vi "Sensor information.vi"(8 "error in (no error)":errorcluster, 10 "Table":i32(listbox)) -> (0 "error in (no error) 2":errorcluster)   [LabVIEW 2015]
uses:
  Control Button/Exit.ctl
  Control Button/Save.ctl
  <vilib>/Utility/miscctls.llb/LVRowAndColumnTypeDef.ctl
  Control Button/Delete.ctl
panel:
  out "Row":i32
  out "subarray":string[](array[string])
  in  "Delete":T1
  in  "stop":T2
  in  "Save Button":T3
  out "Active Cell:Active Cell":T4
  # "Sensor Information"
  # "Sensor Name & Unit"
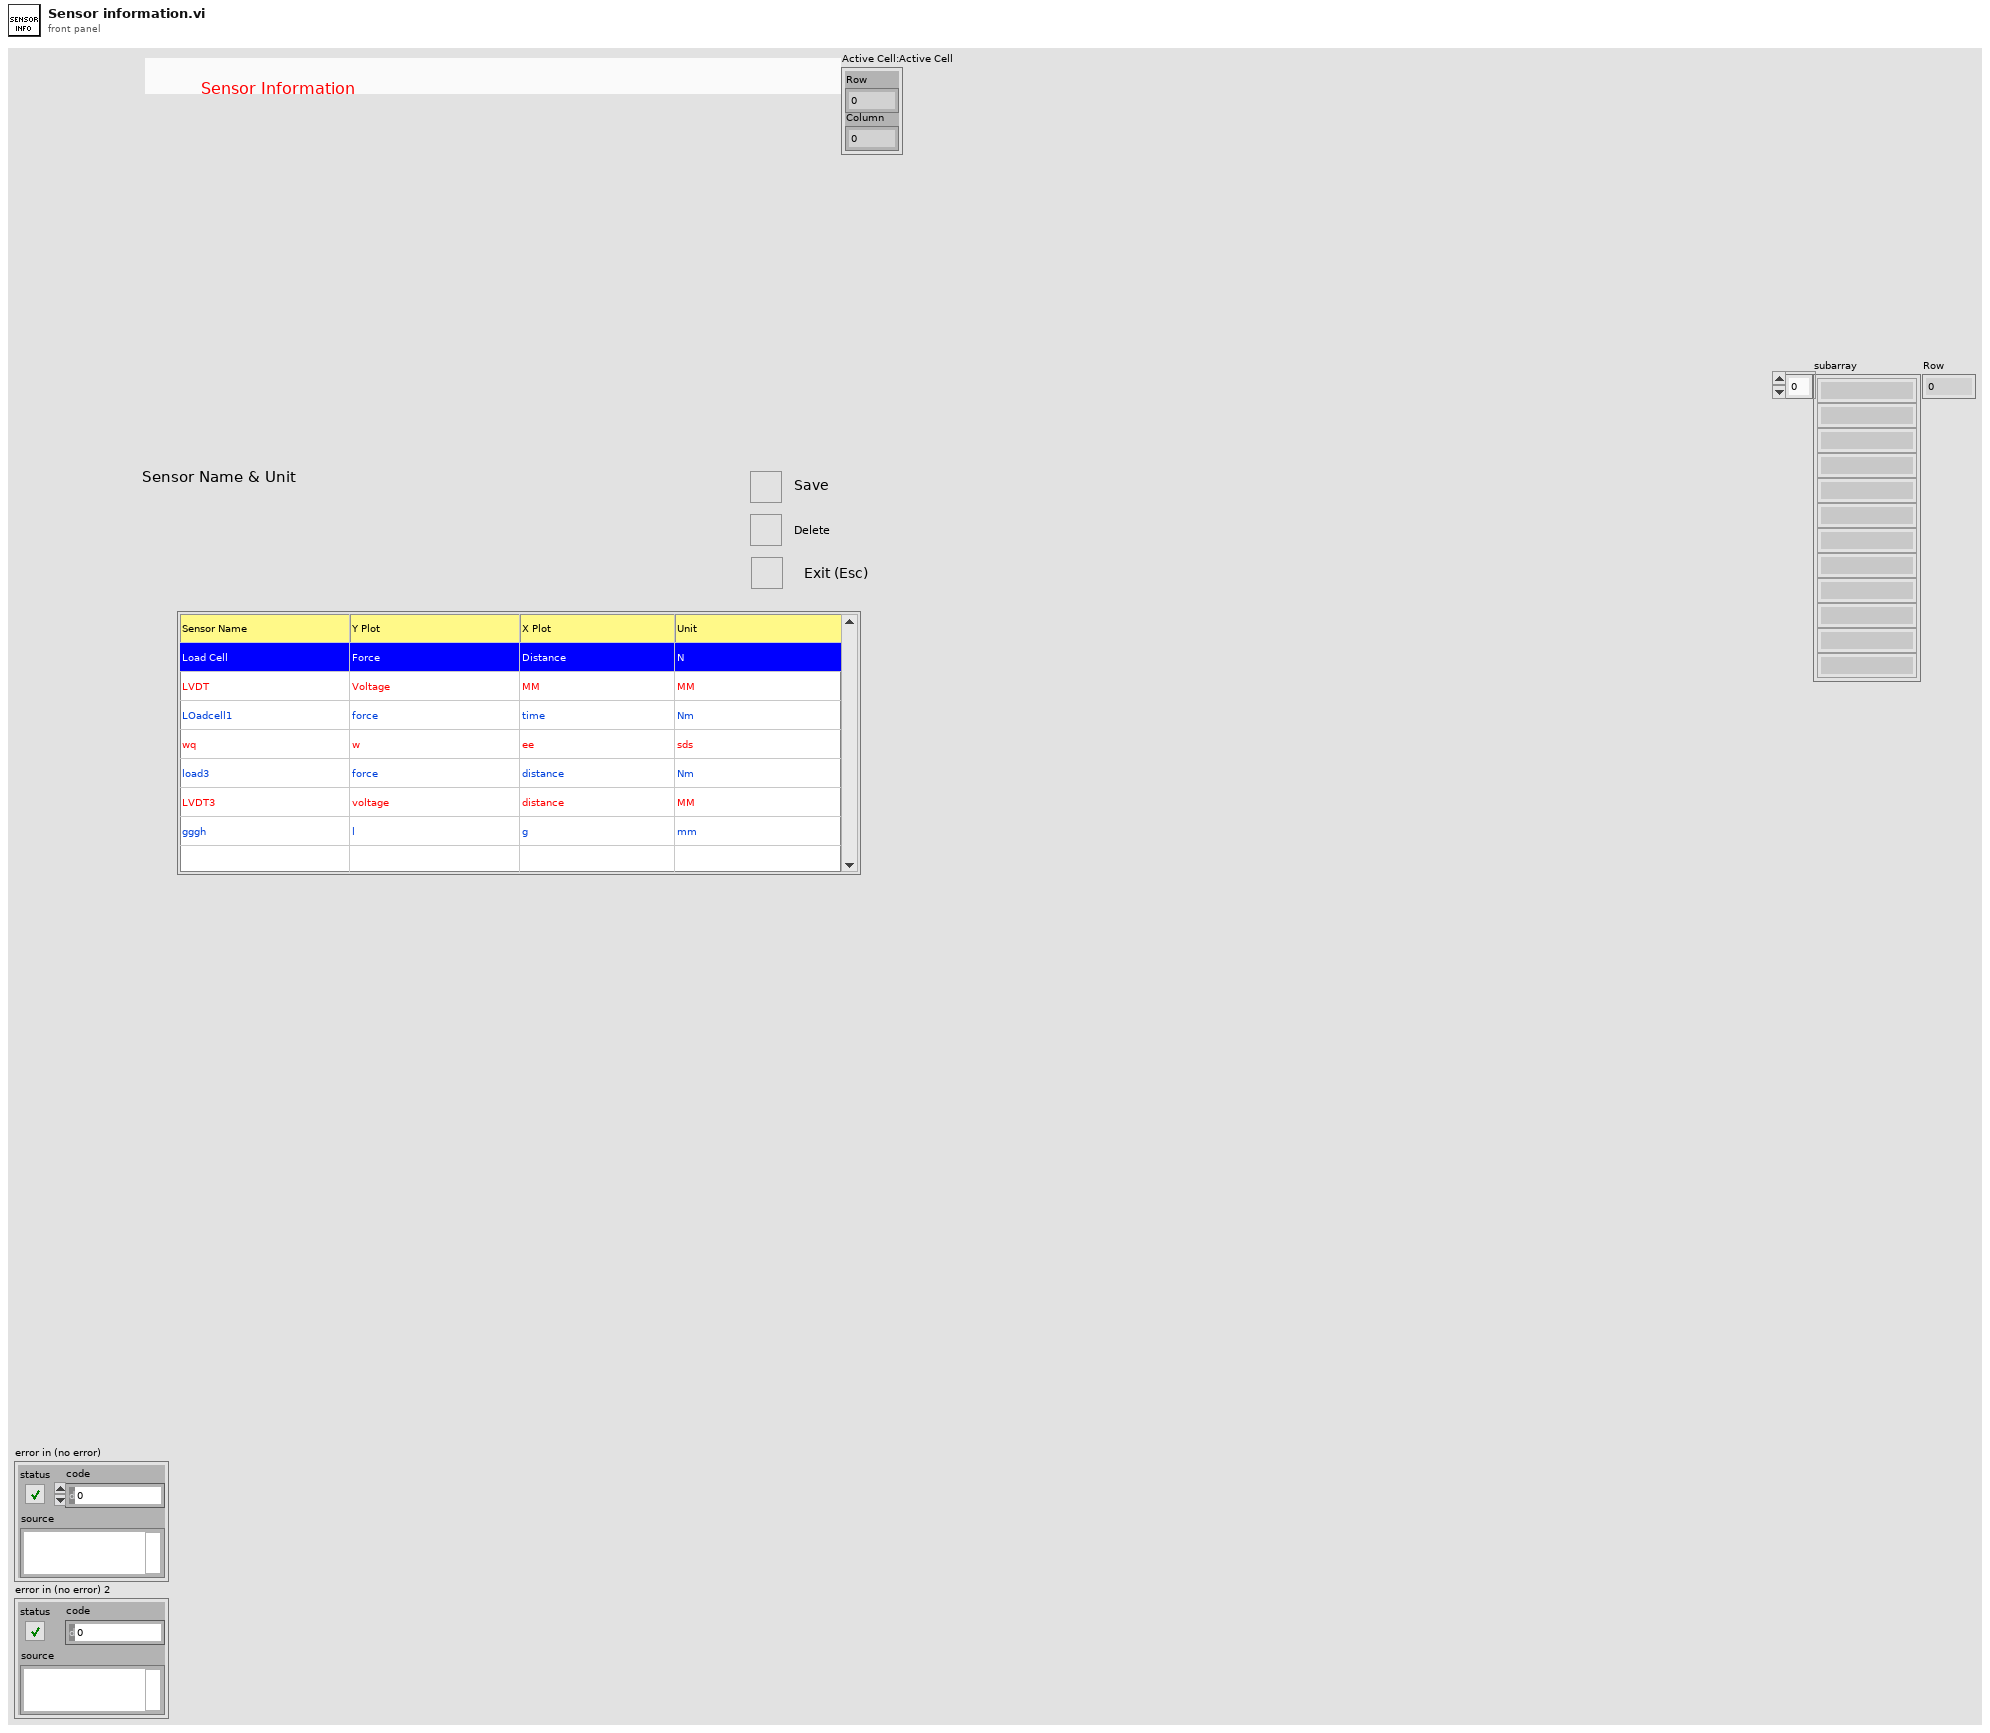
[diagram p1: front panel]
types:
  T1 = typedef "Delete.ctl" = bool
  T2 = typedef "Exit.ctl" = bool
  T3 = typedef "Save.ctl" = bool
  T4 = typedef "LVRowAndColumnTypeDef.ctl" = cluster{"Row":i32, "Column":i32}
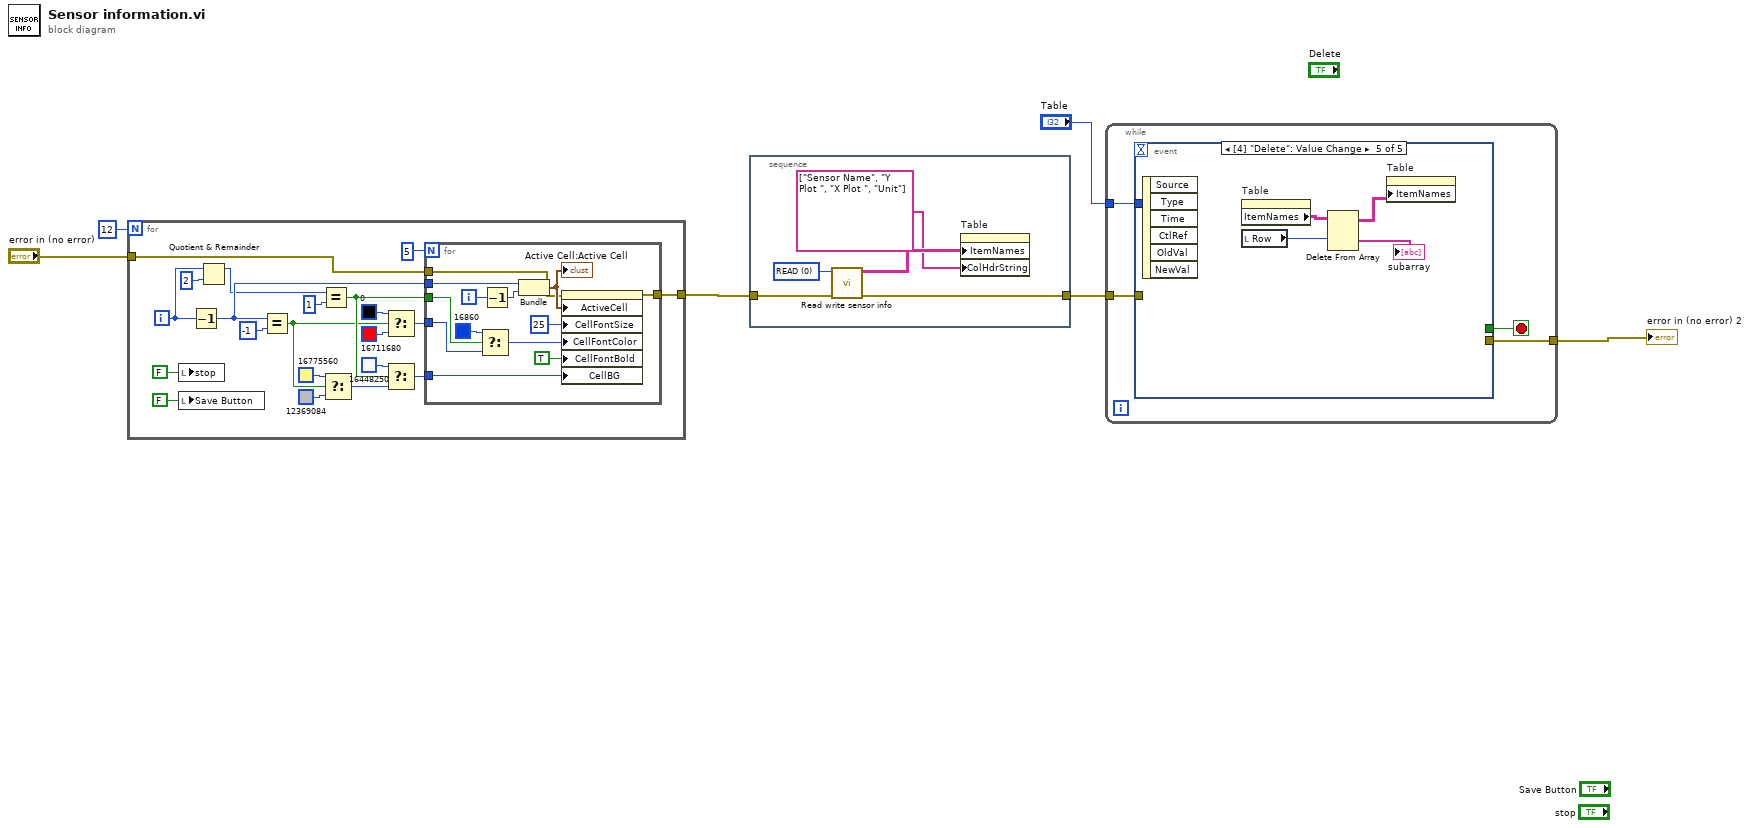
[diagram p0: block diagram]
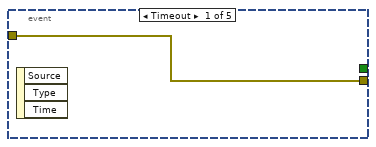
[diagram p2: hidden frame]
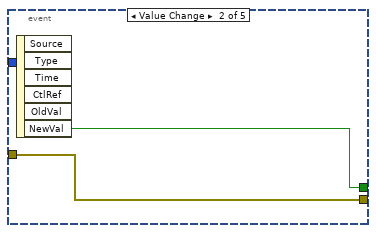
[diagram p3: hidden frame]
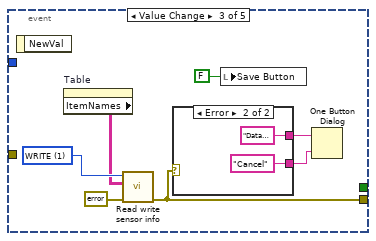
[diagram p4: hidden frame]
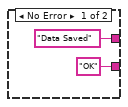
[diagram p5: hidden frame]
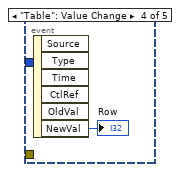
[diagram p6: hidden frame]
diagram:
  n1 = for {
    N: 12 -> [_]
    tunnel: [w10] -> w3
    tunnel: "error in (no error)" -> [w9]
    i -> [w22]
    n2 = local write "stop"(FALSE ("stop")) -> ()
    n3 = local write "Save Button"(FALSE ("Save Button")) -> ()
    n4 = Decrement(x=w22) -> (x-1=w20:i32)
    n5 = Quotient & Remainder(x=w22, y=2) -> (x-y*floor(x/y)=w16:i32)  [unwired: 1 out]
    n6 = Equal?(x=w20, y=-1) -> (x = y?=w13:bool)
    n7 = Equal?(x=w16, y=1) -> (x = y?=w15:bool)
    n8 = Select(t=u32 16775560 ("Color Box"), s=w13, f=u32 12369084 ("Color Box")) -> (s? t:f=w17:u32)
    n9 = Select(t=u32 0 ("Color Box"), s=w13, f=u32 16711680 ("Color Box")) -> (s? t:f=w11:u32)
    n10 = Select(t=u32 16448250 ("Color Box"), s=w15, f=w17) -> (s? t:f=w23:u32)
    n11 = for {
      N: 5 -> [_]
      tunnel: w23 -> [w35]
      tunnel: w20 -> [w39]
      tunnel: w15 -> [w32]
      tunnel: w11 -> [w31]
      tunnel: [w29] -> w10
      tunnel: w9 -> [w28]
      i -> [w38]
      n12 = Select(t=u32 16860 ("Color Box"), s=w32, f=w31) -> (s? t:f=w30:u32)
      n13 = Decrement(x=w38) -> (x-1=w34:i32)
      n14 = Bundle(w39, w34) -> (w37:cluster{i32, i32})  [unwired: 1 in]
      "Active Cell:Active Cell" <- w37
      n15 = property on="Table" class="MCListbox (strict)"(error in=w28, "ActiveCell"=w37, "CellFontSize"=u32 25 ("Active Cell:Cell Font:Size"), "CellFontColor"=w30, "CellFontBold"=TRUE ("Active Cell:Cell Font:Bold"), "CellBG"=w35) -> (error out=w29:errorcluster)  [unwired: 1 in, 1 out]
    }
  }
  n16 = stacked-sequence {
    tunnel: [w41] -> w6
    tunnel: w3 -> [w44]
    frame #0 {
      w45 = u16 0 items=["READ", "WRITE"] ("Read/Write")
      n17 = call "Read write sensor info.vi"("error in (no error)"=w44, "Read/Write"=w45) -> ("error out"=w41:errorcluster, "Table Control out"=w43:string[][])  [unwired: 8 in]
      n18 = property on="Table" class="MCListbox (strict)"("ItemNames"=w43, "ColHdrString"=string[] ["Sensor Name", "Y Plot ", "X Plot ", "Unit"] ("Table Control")) -> ()  [unwired: 2 in, 2 out]
    }
  }
  n19 = while {
    tunnel: w6 -> [w49]
    tunnel: [w48] -> w5
    tunnel: "Table" -> [w46]
    stop <- w47 stop-if-true
    n20 = event shown="[4] \"Delete\": Value Change" {
      selector: _ -> [_ _ _ _ _]
      dyn-events: _ -> [_ _ _ _ _]
      timeout: _ -> [_ _ _ _ _]
      tunnel: w49 -> [w50 w51 _ _ _]
      tunnel: [w50 w51 w56 _ _] -> w48
      tunnel: [_ w52 _ _ _] -> w47
      tunnel: w46 -> [_ _ _ _ _]
      event Timeout {
        n21 = event-data() -> ()  [unwired: 1 in, 3 out]
      }
      event Value Change {
        n22 = event-data() -> ("NewVal"=w52:T2)  [unwired: 1 in, 5 out]
      }
      event Value Change {
        w59 = u16 1 items=["READ", "WRITE"] ("Read/Write")
        n23 = event-data() -> ()  [unwired: 1 in, 1 out]
        n24 = property on="Table" class="MCListbox (strict)"() -> ("ItemNames"=w53:string[][])  [unwired: 2 in, 2 out]
        n25 = call "Read write sensor info.vi"("error in (no error)"=errorcluster {"status"=FALSE, "code"=0, "source"=""}, "Table Control in"=w53, "Read/Write"=w59) -> ("error out"=w56:errorcluster)  [unwired: 7 in, 1 out]
        n26 = case shown="Error" w56 {
          tunnel: ["Data Saved" ("message") "Data Not Saved,Check The File Path" ("message")] -> w55
          tunnel: ["OK" ("button name (\"OK\")") "Cancel" ("button name (\"OK\")")] -> w54
          frame No Error {
          }
          frame Error {
          }
        }
        n27 = local write "Save Button"(FALSE ("Save Button")) -> ()
        n28 = One Button Dialog(message=w55, button name ("OK")=w54) -> ()  [unwired: 1 out]
      }
      event "Table": Value Change {
        n29 = event-data() -> ("NewVal"=→"Row":i32)  [unwired: 1 in, 5 out]
      }
      event Value Change {
        n30 = event-data() -> ()  [unwired: 1 in, 6 out]
        n31 = property on="Table" class="MCListbox (strict)"() -> ("ItemNames"=w68:string[][])  [unwired: 2 in, 2 out]
        n32 = local read "Row"() -> (w66:i32)
        n33 = Delete From Array(array=w68, index (row)=w66) -> (deleted portion=→"subarray":string[], array with subset deleted=w65:string[][])  [unwired: 2 in]
        n34 = property on="Table" class="MCListbox (strict)"("ItemNames"=w65) -> ()  [unwired: 2 in, 2 out]
      }
    }
  }
  "error in (no error) 2" <- w5
